vi "InitialiseProbeplan.vi"(8 "error in (no error)":errorcluster, 10 "Simulation":bool, 11 "ProbeStationControl in":refnum<class "ProbeStationControl.lvclass">) -> (0 "error out":errorcluster, 3 "ProbeStationControl out":refnum<class "ProbeStationControl.lvclass">)   [LabVIEW 2018]
doc: "General utility to initialise, generate, test and execute probe plans."
uses:
  ProbePlanParams.vi
  InstrControl/ProbeStationControl/ProbeStationControl.lvclass
  general_VIs/globals/QC_MeasurementSetup.vi
panel:
  in  "Continue":bool
  in  "New Sensor":bool
  in  "Single Needle":bool
  in  "Probe Card Channels":i32=32
  in  "Strip No.":u16(ring)
  out "Probeplan:":string
  in  "Region":u16(ring)
  in  "Chuck":bool caption="Chuck\nDOWN"
  in  "New Button":bool
  in  "Jump Button":bool
  out "Chuck Up/Down check":bool
  # "Probeplan"
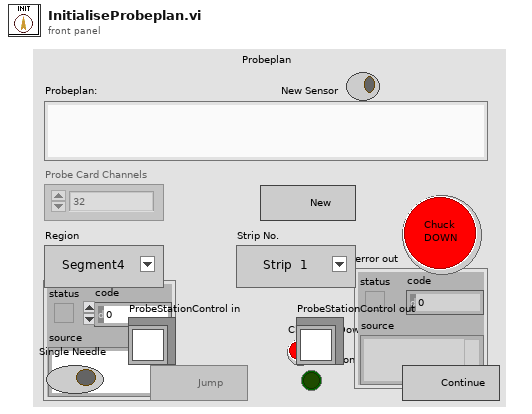
[diagram p1: front panel]
types:
  T1 = cluster{"Strip Number OUT":i32, "X0":i32, "Y0":i32, "X1":i32, "Y1":i32, "Xref":dbl, "Yref":dbl, "ProbePlan type":u32, "Inner pads offset":ext, "Outer pads offset":ext, "l_inner":ext, "l_outer":ext, "strip numbering":u16, "Device Orientation":ext, "Stagger offset":i32, "Yoffset":dbl, "Strip pitch":dbl, "Fiducail separation":dbl, "Radius":ext, "Relative strip angles":dbl, "Probeplan description":string, "ProbePlan array":cluster{"Region":string, "ProbePoints":cluster{"X":dbl, "Y":dbl, "Label":string, "CardViable?":bool}[]}[], "Test ProbePoints":cluster{"Regions Enabled":bool[], "From index":u32[], "To index":u32[], "Strip length [cm]":dbl[]}}
  T2 = cluster{"Bias Supply":refnum<class "SupplyControl.lvclass">, "SMU":refnum<class "SupplyControl.lvclass">, "LCR":refnum<class "LCRControl.lvclass">, "ProbeStation":refnum<class "ProbeStationControl.lvclass">, "Arduino":refnum<class "ArduinoControl.lvclass">, "Measurement switch":refnum<class "Switching.lvclass">, "Probe Card Channels":i32, "Bias Voltage [V]":dbl, "First strip":i32, "Last strip":i32, "Base Voltage [V]":dbl, "Base Ramp Step [V]":dbl, "Base Ramp Interval [ms]":u32, "High Voltage [V]":dbl, "High Ramp Step [V]":dbl, "High Ramp Interval [ms]":u32, "AC frequency [Hz]":i32, "AC amplitude [V]":dbl, "RC Configuration":u16, "Single Needle":bool, "Temperature Readout":enum16{"Read Arduino", "Enter manually"}, "Fraction of good strips [%]":dbl, "Measurement switch used?":bool, "Matrix X Channels":cluster{"Mux1 C1":i32, "Mux1 C2":i32, "Mux2 C1":i32, "Mux2 C2":i32}, "Pinholes Y/N":bool, "Capacitance Y/N":bool, "Resistance Y/N":bool, "Bias Supply Name":string, "SMU Name":string, "LCR Name":string}
  T3 = cluster{"Region":string, "ProbePoints":cluster{"X":dbl, "Y":dbl, "Label":string, "CardViable?":bool}[]}[]
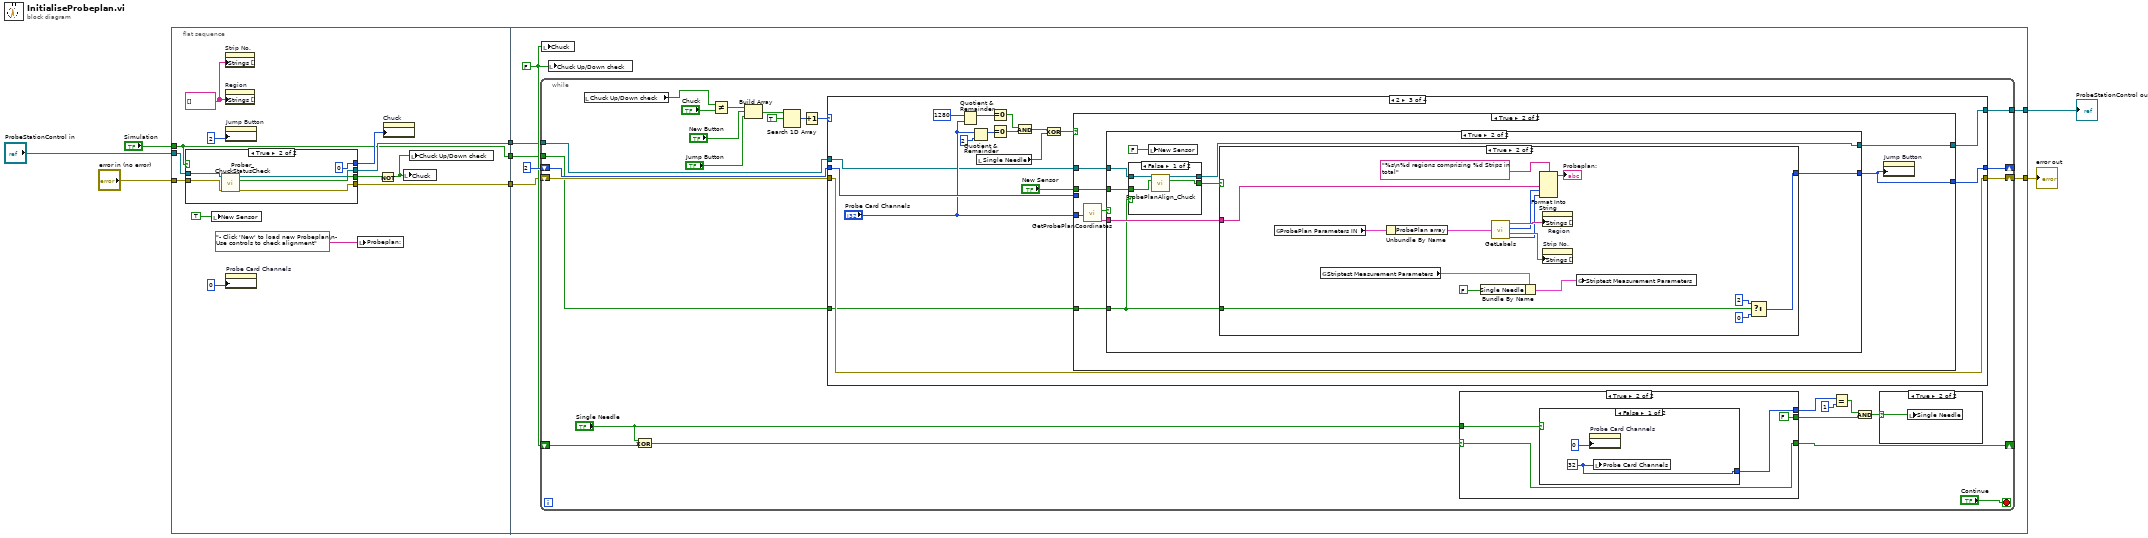
[diagram p0: block diagram]
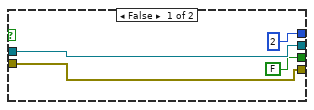
[diagram p2: hidden frame]
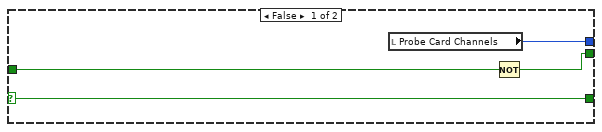
[diagram p4: hidden frame]
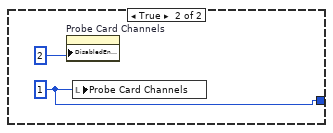
[diagram p5: hidden frame]
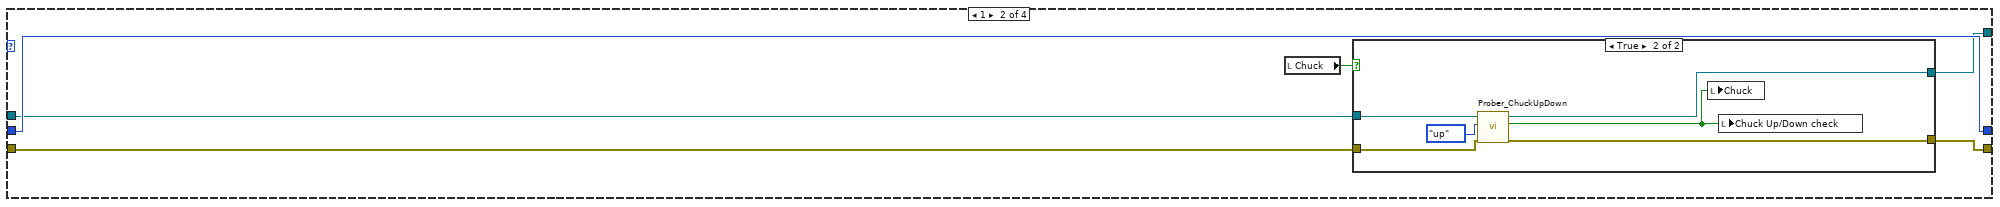
[diagram p7: hidden frame]
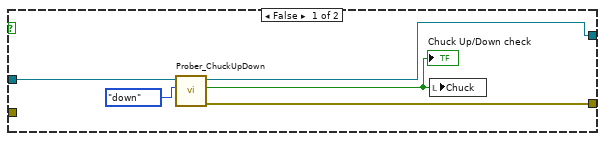
[diagram p8: hidden frame]
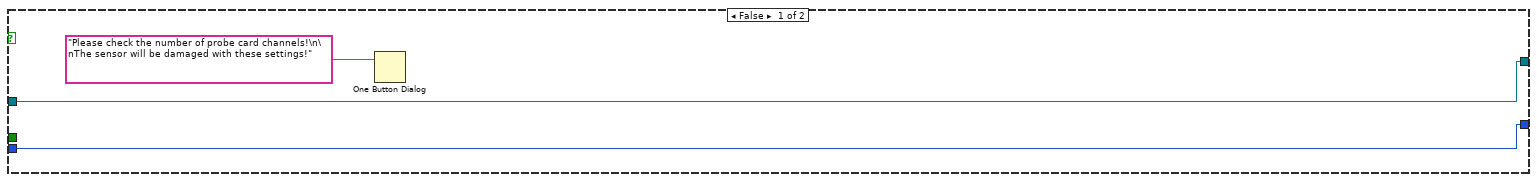
[diagram p9: hidden frame]
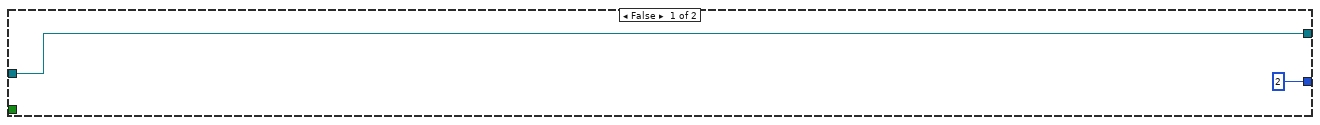
[diagram p10: hidden frame]
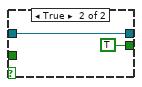
[diagram p11: hidden frame]
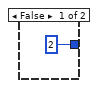
[diagram p12: hidden frame]
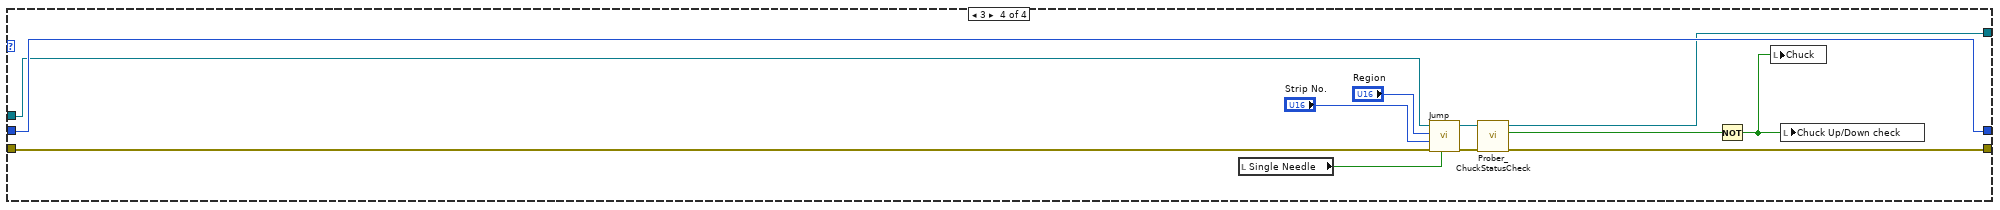
[diagram p13: hidden frame]
diagram:
  n1 = flat-sequence {
    tunnel: "ProbeStationControl in" -> [w15]
    tunnel: [w11] -> w5
    tunnel: "error in (no error)" -> [w13]
    tunnel: [w12] -> w4
    tunnel: "Simulation" -> [w9]
    tunnel: [w9] -> w1
    tunnel: w5 -> [w36]
    tunnel: [w35] -> w7
    tunnel: w4 -> [w34]
    tunnel: [w33] -> w3
    tunnel: w1 -> [w32]
    frame #0 {
      w19 = string[] []
      n2 = case shown="True" w9 {
        tunnel: [FALSE ("Chuck at CONTACT?") w31] -> w17
        tunnel: w15 -> [w24 w30]
        tunnel: w13 -> [w25 w29]
        tunnel: [w25 w28] -> w12
        tunnel: [w24 w27] -> w11
        tunnel: [2 0] -> w10
        frame False {
        }
        frame True {
          n3 = call-dynamic "Prober_ChuckStatusCheck.vi"("error in (no error)"=w29, "ProbeStationControl in"=w30) -> ("error out"=w28:errorcluster, "Chuck at CONTACT?"=w31:bool, "ProbeStationControl out"=w27:refnum<class "ProbeStationControl.lvclass">)  [unwired: 7 in]
        }
      }
      n4 = local write "New Sensor"(TRUE) -> ()
      n5 = property on="Strip No." class="Ring (strict)"("Strings []"=w19) -> ()  [unwired: 2 in, 2 out]
      n6 = property on="Region" class="Ring (strict)"("Strings []"=w19) -> ()  [unwired: 2 in, 2 out]
      n7 = property on="Jump Button" class="Bool"("DisabledEnum"=2) -> ()  [unwired: 2 in, 2 out]
      n8 = property on="Probe Card Channels" class="DigNum (strict)"("DisabledEnum"=0) -> ()  [unwired: 2 in, 2 out]
      n9 = local write "Probeplan:"("- Click 'New' to load new Probeplan\n- Use controls to check alignment") -> ()
      n10 = Not(x=w17) -> (.not. x?=w16:bool)
      n11 = property on="Chuck" class="Bool (strict)"("DisabledEnum"=w10) -> ()  [unwired: 2 in, 2 out]
      n12 = local write "Chuck"(w16) -> ()
      n13 = local write "Chuck Up/Down check"(w16) -> ()
    }
    frame #1 {
      w37 = FALSE
      n14 = while {
        shift-right: [w57] -> _
        shift-left: 2 -> [w58]
        shift-right: [w45] -> _
        shift-left: w37 -> [w46]
        tunnel: w36 -> [w43]
        tunnel: [w42] -> w35
        shift-right: [w40] -> w33
        shift-left: w34 -> [w41]
        tunnel: w32 -> [w39]
        stop <- "Continue" stop-if-true
        n15 = local read "Chuck Up/Down check"() -> (w56:bool)
        n16 = Exclusive Or(1:w46, 2:"Single Needle") -> (0:w48:bool)
        n17 = Not Equal?(x=w56, y="Chuck") -> (x != y?=w54:bool)
        n18 = Build Array(w54, "New Button", "Jump Button") -> (w63:bool[])
        n19 = Search 1D Array(1D array=w63, element=TRUE) -> (index of element=w64:i32)  [unwired: 1 in]
        n20 = Increment(x=w64) -> (x+1=w59:i32)
        n21 = case shown="2" w59 {
          tunnel: w58 -> [w80 w86 w112 w170]
          tunnel: [w80 w86 w114 w170] -> w57
          tunnel: w43 -> [w79 w84 w104 w169]
          tunnel: [w79 w83 w103 w168] -> w42
          tunnel: w41 -> [w78 w81 w99 w164]
          tunnel: [w78 w82 w99 w166] -> w40
          tunnel: w39 -> [_ _ w98 _]
          frame 0, Default {
          }
          frame 1 {
            n22 = local read "Chuck"() -> (w85:bool)
            n23 = case shown="True" w85 {
              tunnel: w84 -> [w90 w95]
              tunnel: [w88 w94] -> w83
              tunnel: [w87 w93] -> w82
              tunnel: w81 -> [_ w92]
              frame False {
                n24 = call-dynamic "Prober_ChuckUpDown.vi"("Direction"=enum16{"up", "down"}."down", "ProbeStationControl in"=w90) -> ("error out"=w87:errorcluster, "Chuck at CONTACT?"=w91:bool, "ProbeStationControl out"=w88:refnum<class "ProbeStationControl.lvclass">)  [unwired: 7 in]
                "Chuck Up/Down check" <- w91
                n25 = local write "Chuck"(w91) -> ()
              }
              frame True {
                n26 = call-dynamic "Prober_ChuckUpDown.vi"("error in (no error)"=w92, "Direction"=enum16{"up", "down"}."up", "ProbeStationControl in"=w95) -> ("error out"=w93:errorcluster, "Chuck at CONTACT?"=w97:bool, "ProbeStationControl out"=w94:refnum<class "ProbeStationControl.lvclass">)  [unwired: 6 in]
                n27 = local write "Chuck"(w97) -> ()
                n28 = local write "Chuck Up/Down check"(w97) -> ()
              }
            }
          }
          frame 2 {
            n29 = Quotient & Remainder(x=1280, y="Probe Card Channels") -> (x-y*floor(x/y)=w113:i32)  [unwired: 1 out]
            n30 = Quotient & Remainder(x="Probe Card Channels", y=2) -> (x-y*floor(x/y)=w107:i32)  [unwired: 1 out]
            n31 = local read "Single Needle"() -> (w100:bool)
            n32 = Equal To 0?(x=w113) -> (x = 0?=w111:bool)
            n33 = Equal To 0?(x=w107) -> (x = 0?=w106:bool)
            n34 = And(x=w111, y=w106) -> (x .and. y?=w102:bool)
            n35 = Exclusive Or(1:w100, 2:w102) -> (0:w101:bool)
            n36 = case shown="True" w101 {
              tunnel: "Probe Card Channels" -> [_ w123]
              tunnel: [w115 w122] -> w114
              tunnel: w112 -> [w115 _]
              tunnel: "New Sensor" -> [_ w121]
              tunnel: w104 -> [w116 w120]
              tunnel: [w116 w119] -> w103
              tunnel: w98 -> [_ w118]
              frame False {
                n37 = One Button Dialog(message="Please check the number of probe card channels!\n\nThe sensor will be damaged with these settings!") -> ()  [unwired: 1 in, 1 out]
              }
              frame True {
                n38 = call "GetProbePlanCoordinates.vi"("Probe Card Channels"=w123) -> ("file path"=w124:string, "OK?"=w125:bool)  [unwired: 1 out]
                n39 = case shown="True" w125 {
                  tunnel: [2 w135] -> w122
                  tunnel: w124 -> [_ w133]
                  tunnel: w121 -> [_ w132]
                  tunnel: w120 -> [w126 w131]
                  tunnel: [w126 w130] -> w119
                  tunnel: w118 -> [_ w128]
                  frame False {
                  }
                  frame True {
                    n40 = case shown="False" w128 {
                      tunnel: [w139 TRUE] -> w134
                      tunnel: w132 -> [w138 _]
                      tunnel: w131 -> [w137 w140]
                      tunnel: [w136 w140] -> w130
                      frame False {
                        n41 = call "ProbePlanAlign_Chuck.vi"("New Sensor"=w138, "ProbeStationControl in"=w137) -> ("Accept/Quit"=w139:bool, "ProbeStationControl out"=w136:refnum<class "ProbeStationControl.lvclass">)  [unwired: 8 in]
                      }
                      frame True {
                      }
                    }
                    n42 = local write "New Sensor"(FALSE) -> ()
                    n43 = case shown="True" w134 {
                      tunnel: [2 w146] -> w135
                      tunnel: w133 -> [_ w144]
                      tunnel: w128 -> [_ w148]
                      frame False {
                      }
                      frame True {
                        n44 = global read "ProbePlanParams.vi" "ProbePlan Parameters IN"() -> (w158:T1)
                        n45 = global read "QC_MeasurementSetup.vi" "Striptest Measurement Parameters"() -> (w151:T2)
                        n46 = Unbundle By Name(w158) -> ("ProbePlan array"=w157:T3)
                        n47 = Bundle By Name(cluster=w151, "Single Needle"=FALSE) -> (w150:T2)
                        n48 = call "GetLabels.vi"("Array"=w157) -> ("Region Labels"=w155:string[], "No. of regions"=w145:i32, "Strip Labels"=w156:string[], "No. of Points"=w154:i32)
                        n49 = Format Into String(format string="%s\n%d regions comprising %d Strips in total", w144, w145, w154) -> (resulting string=→"Probeplan:":string)  [unwired: 2 in, 1 out]
                        n50 = property on="Region" class="Ring (strict)"("Strings []"=w155) -> ()  [unwired: 2 in, 2 out]
                        n51 = property on="Strip No." class="Ring (strict)"("Strings []"=w156) -> ()  [unwired: 2 in, 2 out]
                        n52 = global write "QC_MeasurementSetup.vi" "Striptest Measurement Parameters"(w150) -> ()
                        n53 = Select(t=2, s=w148, f=0) -> (s? t:f=w146:i32)
                      }
                    }
                  }
                }
                n54 = property on="Jump Button" class="Bool"("DisabledEnum"=w122) -> ()  [unwired: 2 in, 2 out]
              }
            }
          }
          frame 3 {
            n55 = local read "Single Needle"() -> (w161:bool)
            n56 = call "Jump.vi"("Single Needle"=w161, "Error In"=w164, "Strip No."="Strip No.", "Region"="Region", "ProbeStationControl in"=w169) -> ("Error Out"=w165:errorcluster, "ProbeStationControl out"=w167:refnum<class "ProbeStationControl.lvclass">)  [unwired: 5 in]
            n57 = call-dynamic "Prober_ChuckStatusCheck.vi"("error in (no error)"=w165, "ProbeStationControl in"=w167) -> ("error out"=w166:errorcluster, "Chuck at CONTACT?"=w160:bool, "ProbeStationControl out"=w168:refnum<class "ProbeStationControl.lvclass">)  [unwired: 7 in]
            n58 = Not(x=w160) -> (.not. x?=w159:bool)
            n59 = local write "Chuck"(w159) -> ()
            n60 = local write "Chuck Up/Down check"(w159) -> ()
          }
        }
        n61 = case shown="True" w48 {
          selector: w48 -> [w66 w70]
          tunnel: [w68 FALSE] -> w51
          tunnel: [w69 w72] -> w49
          tunnel: "Single Needle" -> [w67 w71]
          tunnel: [w66 w70] -> w45
          frame False {
            n62 = local read "Probe Card Channels"() -> (w69:i32)
            n63 = Not(x=w67) -> (.not. x?=w68:bool)
          }
          frame True {
            n64 = case shown="False" w71 {
              tunnel: [w74 w77] -> w72
              frame False {
                w74 = 32
                n65 = property on="Probe Card Channels" class="DigNum (strict)"("DisabledEnum"=0) -> ()  [unwired: 2 in, 2 out]
                n66 = local write "Probe Card Channels"(w74) -> ()
              }
              frame True {
                w77 = 1
                n67 = property on="Probe Card Channels" class="DigNum (strict)"("DisabledEnum"=2) -> ()  [unwired: 2 in, 2 out]
                n68 = local write "Probe Card Channels"(w77) -> ()
              }
            }
          }
        }
        n69 = Equal?(x=w49, y=1) -> (x = y?=w52:bool)
        n70 = And(x=w52, y=w51) -> (x .and. y?=w50:bool)
        n71 = case shown="True" w50 {
          selector: w50 -> [_ w65]
          frame False {
          }
          frame True {
            n72 = local write "Single Needle"(w65) -> ()
          }
        }
      }
      n73 = local write "Chuck"(w37) -> ()
      n74 = local write "Chuck Up/Down check"(w37) -> ()
    }
  }
  "ProbeStationControl out" <- w7
  "error out" <- w3
